vi "_TEST_locker.vi"   [LabVIEW 2017]
uses:
  ObjectCacherAPI.lvlib
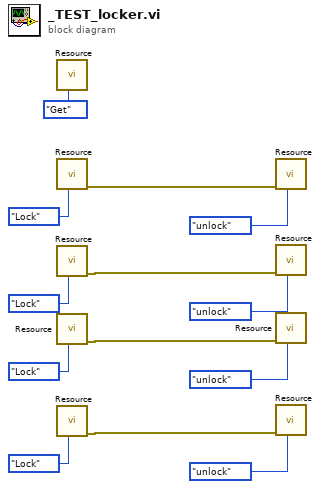
[diagram p0: block diagram]
diagram:
  n1 = call "Resource.vi"("action"=enum16{"Get", "Lock", "unlock"}."Get") -> ()  [unwired: 8 in, 3 out]
  n2 = call "Resource.vi"("action"=enum16{"Get", "Lock", "unlock"}."Lock") -> ("error out"=w10:errorcluster)  [unwired: 8 in, 2 out]
  n3 = call "Resource.vi"("action"=enum16{"Get", "Lock", "unlock"}."Lock") -> ("error out"=w9:errorcluster)  [unwired: 8 in, 2 out]
  n4 = call "Resource.vi"("action"=enum16{"Get", "Lock", "unlock"}."Lock") -> ("error out"=w4:errorcluster)  [unwired: 8 in, 2 out]
  n5 = call "Resource.vi"("action"=enum16{"Get", "Lock", "unlock"}."Lock") -> ("error out"=w3:errorcluster)  [unwired: 8 in, 2 out]
  n6 = call "Resource.vi"("action"=enum16{"Get", "Lock", "unlock"}."unlock", "error in (no error)"=w10) -> ()  [unwired: 7 in, 3 out]
  n7 = call "Resource.vi"("action"=enum16{"Get", "Lock", "unlock"}."unlock", "error in (no error)"=w9) -> ()  [unwired: 7 in, 3 out]
  n8 = call "Resource.vi"("action"=enum16{"Get", "Lock", "unlock"}."unlock", "error in (no error)"=w4) -> ()  [unwired: 7 in, 3 out]
  n9 = call "Resource.vi"("action"=enum16{"Get", "Lock", "unlock"}."unlock", "error in (no error)"=w3) -> ()  [unwired: 7 in, 3 out]
